vi "RotateCalc.vi"(6 "Joystick 1X":dbl, 8 "Wheel2":dbl, 9 "Wheel1":dbl) -> (0 "Left angel":dbl, 1 "Right angel":dbl, 2 "Left Speed":dbl, 3 "Right speed":dbl)   [LabVIEW 2011]
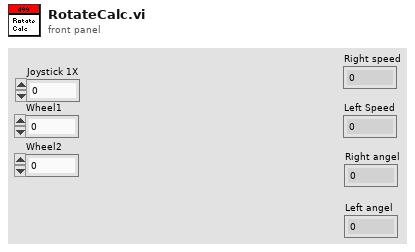
[diagram p1: front panel]
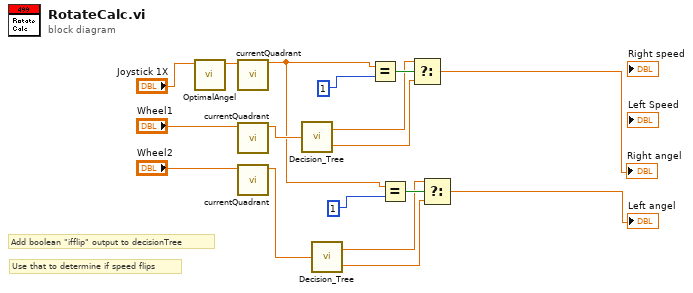
[diagram p0: block diagram]
diagram:
  # "Use that to determine if speed flips"
  # "Add boolean \"ifflip\" output to decisionTree"
  n1 = call "OptimalAngel.vi"("Joystick X"="Joystick 1X") -> ("Angel"=w14:dbl)  [unwired: 10 in]
  n2 = call "currentQuadrant.vi"("Wheel"=w14) -> ("Quadrent"=w3:dbl)  [unwired: 10 in]
  n3 = call "currentQuadrant.vi"("Wheel"="Wheel1") -> ("Quadrent"=w10:dbl)  [unwired: 10 in]
  n4 = call "currentQuadrant.vi"("Wheel"="Wheel2") -> ("Quadrent"=w2:dbl)  [unwired: 10 in]
  n5 = call "Decision_Tree.vi"("Numeric"=w10) -> ("Case 1"=w9:dbl, "Case 2"=w8:dbl)
  n6 = call "Decision_Tree.vi"("Numeric"=w2) -> ("Case 1"=w5:dbl, "Case 2"=w4:dbl)
  n7 = Equal?(x=w3, y=1) -> (x = y?=w12:bool)
  n8 = Equal?(x=w3, y=1) -> (x = y?=w6:bool)
  n9 = Select(t=w9, s=w12, f=w8) -> (s? t:f=→"Right angel":dbl)
  n10 = Select(t=w5, s=w6, f=w4) -> (s? t:f=→"Left angel":dbl)
